vi "FitImageToDisplay.vi"(9 "Image Control Reference":refnum<vi>, 10 "Image":T1) -> (3 "Image (dup)":T1)   [LabVIEW 2016]
uses:
  <vilib>/vision/Image Controls.llb/IMAQ Image.ctl
panel:
  out "error out":errorcluster
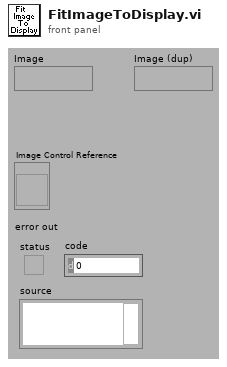
[diagram p1: front panel]
types:
  T1 = typedef "IMAQ Image.ctl" = refnum<image>
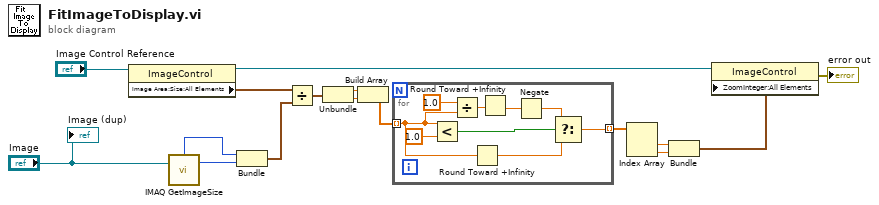
[diagram p0: block diagram]
diagram:
  n1 = property class="ImageControl"(reference="Image Control Reference") -> (reference out=w13:refnum<vi>, "Image Area:Size:All Elements"=w10:cluster{"Width":u32, "Height":u32})  [unwired: 1 in, 1 out]
  n2 = call "IMAQ GetImageSize"("Image"="Image") -> ("Y Resolution"=w14:i32, "X Resolution"=w15:i32)  [unwired: 3 in, 1 out]
  n3 = Bundle("X Resolution"=w15, "Y Resolution"=w14) -> (w9:cluster{"X Resolution":i32, "Y Resolution":i32})  [unwired: 1 in]
  n4 = Divide(x=w10, y=w9) -> (x/y=w8:cluster{dbl, dbl})
  n5 = Unbundle(w8) -> (w7:dbl, w6:dbl)
  n6 = Build Array(w7, w6) -> (w5:dbl[])
  n7 = for {
    tunnel: w5 -> [w22] mode=indexing
    tunnel: [w17] -> w4 mode=indexing
    n8 = Less?(x=w22, y=1.0) -> (x < y?=w23:bool)
    n9 = Divide(x=1.0, y=w22) -> (x/y=w21:dbl)
    n10 = Round Toward +Infinity(x=w22) -> (ceil(x): smallest int >= x=w19:dbl)
    n11 = Round Toward +Infinity(x=w21) -> (ceil(x): smallest int >= x=w20:dbl)
    n12 = Negate(x=w20) -> (-x=w18:dbl)
    n13 = Select(t=w18, s=w23, f=w19) -> (s? t:f=w17:dbl)
  }
  n14 = Index Array(array=w4) -> (element #1=w2:dbl, element #2=w3:dbl)  [unwired: 2 in]
  n15 = Bundle(w2, w3) -> (w1:cluster{dbl, dbl})  [unwired: 1 in]
  n16 = property class="ImageControl"(reference=w13, "ZoomInteger:All Elements"=w1) -> (error out=→"error out":errorcluster)  [unwired: 1 in, 1 out]
  "Image (dup)" <- "Image"
